vi "Untitled 1.vi"   [LabVIEW 2016]
uses:
  Classes/Workspace/Component/Component Tray.lvclass
  Classes/Workspace/Carrier Tray/Baseplate Tray.lvclass
  Classes/Controller/Controller.lvclass
types:
  T1 = typedef "Controller.lvclass/Controllers.ctl" = cluster{"I-O.lvclass":refnum<class "I-O.lvclass">, "Motion.lvclass":refnum<class "Motion.lvclass">, "Dispenser.lvclass":refnum<class "Dispenser.lvclass">}
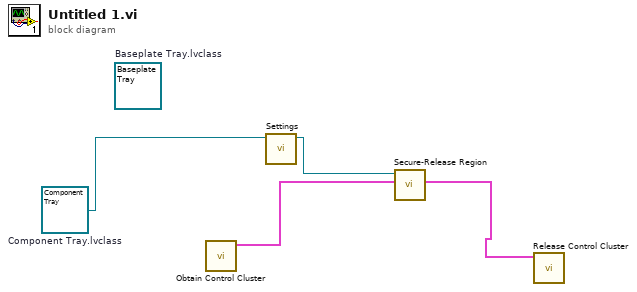
[diagram p0: block diagram]
diagram:
  w1 = refnum<class "Component Tray.lvclass"> refnum  # Component Tray.lvclass
  (unwired) refnum<class "Baseplate Tray.lvclass"> refnum  # Baseplate Tray.lvclass
  n1 = call "Obtain Control Cluster.vi"() -> ("Control Out"=w3:T1)  [unwired: 11 in]
  n2 = call-dynamic "Settings.vi"("Component in"=w1) -> ("Component out"=w4:refnum<class "Component Tray.lvclass">)  [unwired: 9 in, 1 out]
  n3 = call-dynamic "Secure-Release Region.vi"("Control In"=w3, "Component in"=w4) -> ("Control Out"=w2:T1)  [unwired: 7 in, 2 out]
  n4 = call "Release Control Cluster.vi"("output cluster"=w2) -> ()  [unwired: 11 in]
